vi "Motion Done.vi"(8 "error in (no error)":errorcluster, 10 "Axis":i32, 11 ".NET Refnum in":refnum<k24>) -> (0 "error out":errorcluster, 2 "Done":bool)   [LabVIEW 2020, in "ESP301-Driver.lvlib"]
uses:
  ESP301-Driver.lvlib
  Newport.ESP301.CommandInterface
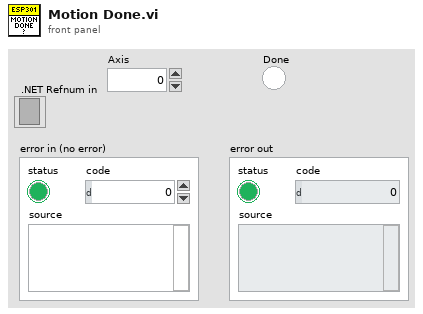
[diagram p1: front panel]
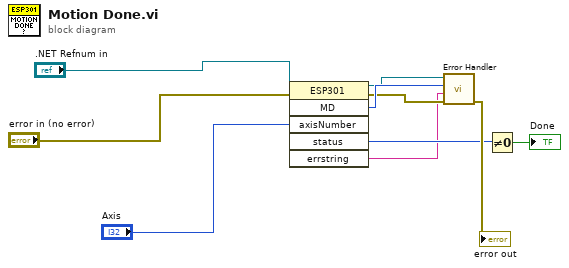
[diagram p0: block diagram]
diagram:
  n1 = invoke class="ESP301" method="MD"(reference=".NET Refnum in", error in="error in (no error)", "axisNumber"="Axis") -> (reference out=w9:refnum<k24>, error out=w3:errorcluster, "MD"=w10:i32, "status"=w6:i32, "errstring"=w1:string)  [unwired: 3 in, 1 out]
  n2 = call "Error Handler.vi"("error in (no error)"=w3, "Message"=w1, "Error Code"=w10, ".NET Refnum in"=w9) -> ("error out"=→"error out":errorcluster)  [unwired: 6 in, 1 out]
  n3 = Not Equal To 0?(x=w6) -> (x != 0?=→"Done":bool)
